vi "Wait on Listener.vi"(8 "error in":errorcluster, 10 "timeout ms (wait forever: -1)":i32, 11 "TCP slave in":refnum<class "TCP Slave.lvclass">) -> (0 "error out":errorcluster, 1 "Timed Out":bool, 2 "connection reference":refnum<data-value>, 3 "TCP slave out":refnum<class "TCP Slave.lvclass">)   [LabVIEW 2012, in "TCP Slave.lvclass"]
doc: "Wrapper for the wait on listener VI, using the listener stored in the slave and an infinite timeout. When a connection is established, the output class will contain the new connection."
uses:
  TCP Slave.lvclass
  Connection.ctl
  TCP Slave.lvclass/TCP Slave.ctl
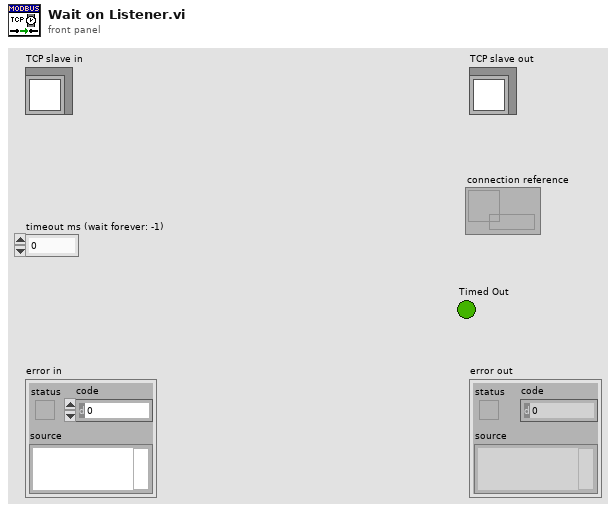
[diagram p1: front panel]
types:
  T1 = typedef "TCP Slave.lvclass/Connection.ctl" = cluster{"Connected?":bool, "IP address":string, "connection error":errorcluster}
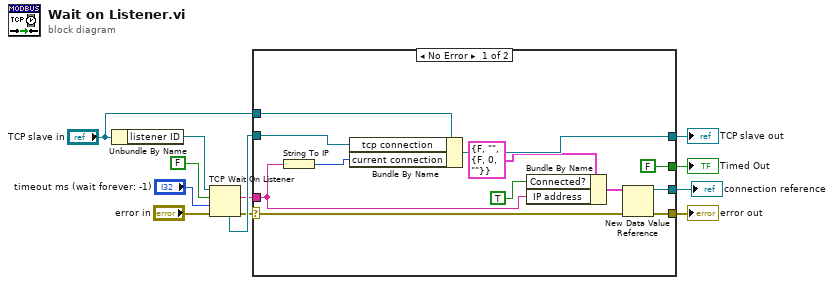
[diagram p0: block diagram]
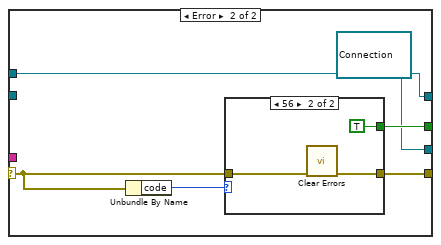
[diagram p2: hidden frame]
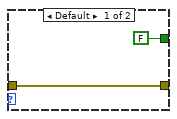
[diagram p3: hidden frame]
diagram:
  n1 = Unbundle By Name("TCP slave in") -> ("listener ID"=w10:refnum<k5>)
  n2 = TCP Wait On Listener(8:"error in", 9:"timeout ms (wait forever: -1)", 10:FALSE ("resolve remote address (T)"), 11:w10) -> (0:w5:errorcluster, 2:w1:string, 4:w9:refnum<k5>)  [unwired: 2 out]
  n3 = case shown="No Error" w5 {
    selector: w5 -> [w20 w29]
    tunnel: "TCP slave in" -> [w24 w26]
    tunnel: w9 -> [w23 _]
    tunnel: [w21 w26] -> w6
    tunnel: [w15 w28] -> w4
    tunnel: [FALSE w27] -> w3
    tunnel: [w19 refnum<data-value> refnum ("data value reference")] -> w2
    tunnel: w1 -> [w14 _]
    frame No Error {
      n4 = String To IP(1:w14) -> (0:w13:u32)
      n5 = Bundle By Name(cluster=w24, "tcp connection"=w23, "current connection"=w13) -> (w21:refnum<class "TCP Slave.lvclass">)
      n6 = Bundle By Name(cluster=T1 {"Connected?"=FALSE, "IP address"="", "connection error"={"status"=FALSE, "code"=0, "source"=""}} ("Connection"), "Connected?"=TRUE, "IP address"=w14) -> (w17:T1)
      n7 = New Data Value Reference(data value=w17, error in=w20) -> (data value reference=w19:refnum<data-value>, error out=w15:errorcluster)
    }
    frame Error {
      n8 = Unbundle By Name(w29) -> ("code"=w30:i32)
      n9 = case shown="56" w30 {
        tunnel: w29 -> [w32 w35]
        tunnel: [w32 w34] -> w28
        tunnel: [FALSE TRUE] -> w27
        frame Default {
        }
        frame 56 {
          n10 = call <vilib>:"Clear Errors.vi"("error in (no error)"=w35) -> ("error out"=w34:errorcluster)  [unwired: 6 in]
        }
      }
    }
  }
  "error out" <- w4
  "Timed Out" <- w3
  "connection reference" <- w2
  "TCP slave out" <- w6
